vi "dvp Vi Get Resolution Mode Sel.vi"(10 "pResolutionModeSel":u32, 11 "handle":u32) -> (2 "pResolutionModeSel out":u32, 3 "function return":u32(ring))   [LabVIEW 2018, in "LabViewDVPCamera.lvlib"]
doc: "LabviewDvp2Api dvpStatus dvpViGetResolutionModeSel(dvpHandle handle, dvpUint32 *pResolutionModeSel);"
uses:
  LabViewDVPCamera.lvlib
  LabViewDVPCamera/LabViewDVPCamera.dll
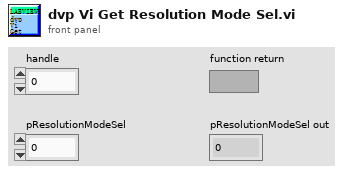
[diagram p1: front panel]
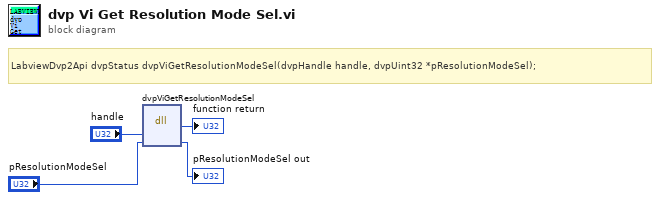
[diagram p0: block diagram]
diagram:
  # "LabviewDvp2Api dvpStatus dvpViGetResolutionModeSel(dvpHandle handle, dvpUint32 *pResolutionModeSel);"
  n1 = dll-call lib="C:/Program Files (x86)/DVP2 Labview cn 64/Sample/LabViewDVPCamera/LabViewDVPCamera.*" fn="dvpViGetResolutionModeSel"("handle"="handle", "pResolutionModeSel"="pResolutionModeSel") -> (→"function return":u32, "pResolutionModeSel"=→"pResolutionModeSel out":u32)  [unwired: 4 in, 2 out]
